vi "Base Init.vi"(9 "Actor":refnum<class "Actor.lvclass">, 10 "Self Alias":string) -> (2 "Actor":refnum<class "Actor.lvclass">)   [LabVIEW 2020, in "jettl.lvlib" / "Actor.lvlib"]
uses:
  Actor.lvlib
  Base Actor/Base Actor.lvclass
  Msg/Msg.lvclass
  Implemented Msgs.ctl
  Attributes.ctl
  Actor/Actor.lvclass
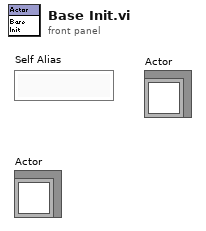
[diagram p1: front panel]
types:
  T1 = typedef "jettl.lvlib/Actor.lvlib/Attributes.ctl" = cluster{"Alias":string, "Address":refnum<user-event>, "Implemented Msgs":T2, "Path":path}
  T2 = typedef "jettl.lvlib/Actor.lvlib/Implemented Msgs.ctl" = set{refnum<class "Msg.lvclass">}
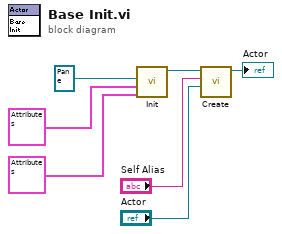
[diagram p0: block diagram]
diagram:
  n1 = call "Init.vi"("Creator Attributes"=T1 {"Alias"="", "Address"=refnum, "Implemented Msgs"={}, "Path"=path ""}, "Self Attributes"=T1 {"Alias"="", "Address"=refnum, "Implemented Msgs"={}, "Path"=path ""}, "Register"=refnum<event-registration> refnum) -> ("Base Actor out"=w4:refnum<class "Base Actor.lvclass">)  [unwired: 8 in]
  n2 = call-dynamic "Create.vi"("Actor"="Actor", "Self Alias"="Self Alias", "Base Actor in"=w4) -> ("Base Actor out"=→"Actor":refnum<class "Base Actor.lvclass">)  [unwired: 8 in]
